vi "Test Sequencer Example.vi"() -> ()   [LabVIEW 2010]
doc: "Car Wash Main VI. Allows setup of multiple wash steps and sim of car position. Shows current step."
uses:
  Sequence Table/Sequence Table Cluster TDef.ctl
  Controls/StateMachineStates_TEST_TDEF.ctl
panel:
  out "error out":errorcluster
  out "input cluster":T1
  in  "Abort":bool
  in  "Start":bool
  in  "Pause":bool
  out "Test Running":bool
  out "Elapsed Time":dbl format="%.2g"
  in  "Test Table":string[][](table)=[[""]]
  out "Current Test":string[](array[string])
  in  "Stop Program":bool
  # "Test Sequence Configuration"
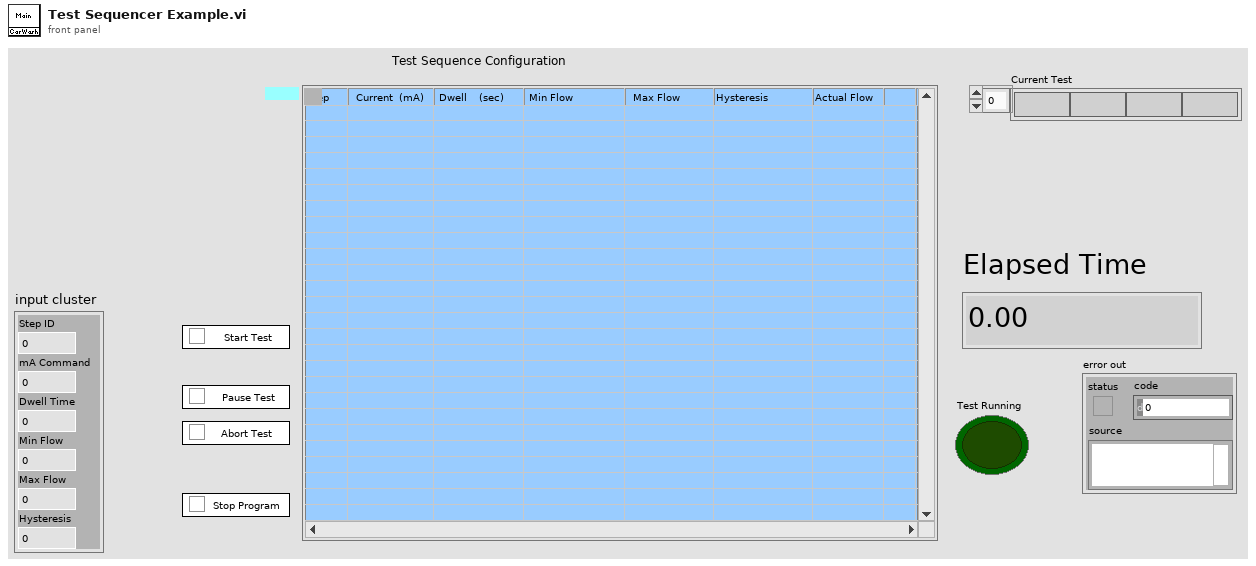
[diagram p1: front panel]
types:
  T1 = typedef "Sequence Table Cluster TDef.ctl" = cluster{"Step ID":i32, "mA Command":dbl, "Dwell Time":dbl, "Min Flow":dbl, "Max Flow":dbl, "Hysteresis":dbl}
  T2 = typedef "StateMachineStates_TEST_TDEF.ctl" = enum16{"Initialize", "Start", "Run Position", "Pause", "Resume", "Get Step"}
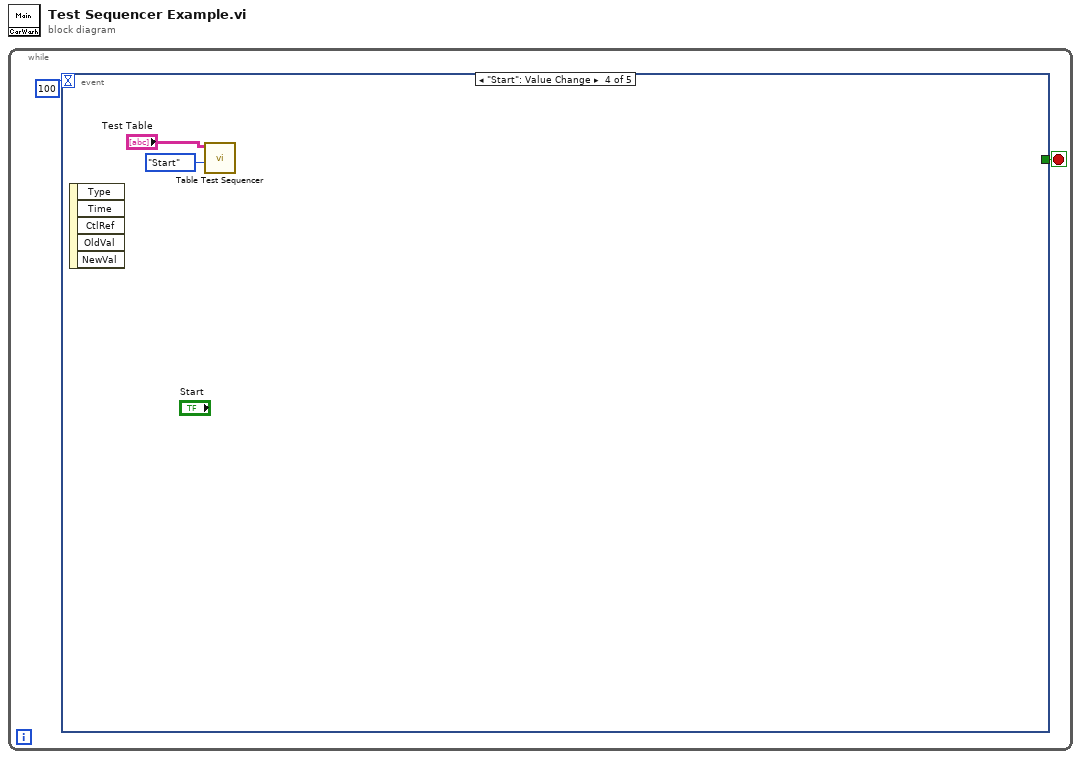
[diagram p0: block diagram]
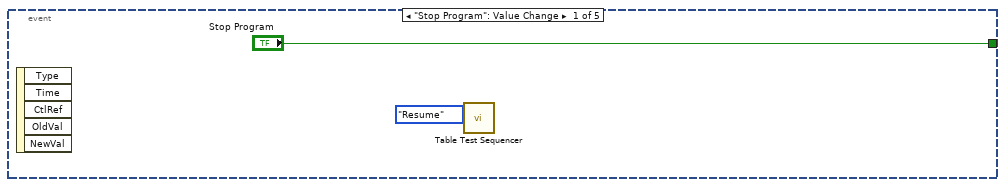
[diagram p2: hidden frame]
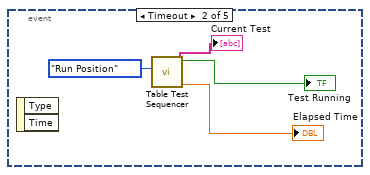
[diagram p3: hidden frame]
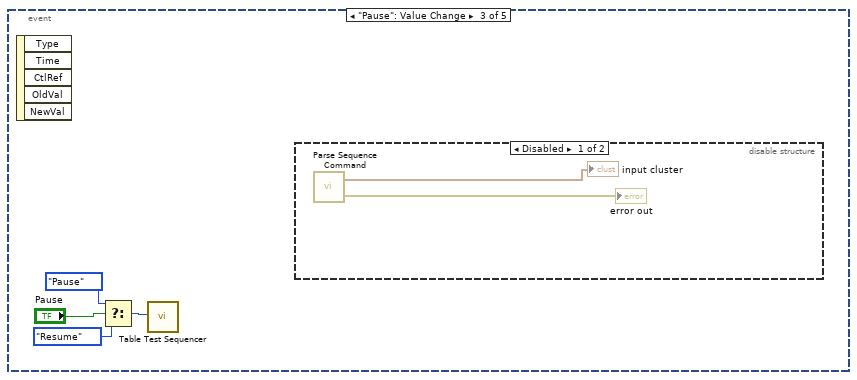
[diagram p4: hidden frame]
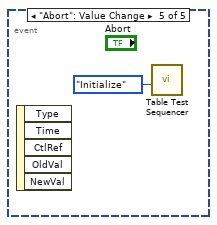
[diagram p6: hidden frame]
diagram:
  n1 = while {
    stop <- w2 stop-if-true
    n2 = event shown="[3] \"Start\": Value Change" {
      selector: _ -> [_ _ _ _ _]
      dyn-events: _ -> [_ _ _ _ _]
      timeout: 100 -> [_ _ _ _ _]
      tunnel: ["Stop Program" _ _ _ _] -> w2
      event "Stop Program": Value Change {
        n3 = event-data() -> ()  [unwired: 1 in, 5 out]
        n4 = call "Table Test Sequencer.vi"("Action"=StateMachineStates_TEST_TDEF."Resume") -> ()  [unwired: 3 in, 8 out]
      }
      event Timeout {
        n5 = event-data() -> ()  [unwired: 1 in, 2 out]
        n6 = call "Table Test Sequencer.vi"("Action"=StateMachineStates_TEST_TDEF."Run Position") -> ("Current Elapsed"=→"Elapsed Time":dbl, "Test Running"=→"Test Running":bool, "Current Test"=→"Current Test":string[])  [unwired: 3 in, 5 out]
      }
      event "Pause": Value Change {
        n7 = event-data() -> ()  [unwired: 1 in, 5 out]
        n8 = Select(t=StateMachineStates_TEST_TDEF."Pause" ("Action"), s="Pause", f=StateMachineStates_TEST_TDEF."Resume") -> (s? t:f=w9:T2)
        n9 = call "Table Test Sequencer.vi"("Action"=w9) -> ()  [unwired: 3 in, 8 out]
        n10 = disable-structure shown="Disabled" {
          frame Disabled {
            n11 = call "Parse Sequence Command.vi"() -> ("error out"=→"error out":errorcluster, "input cluster"=→"input cluster":T1)  [unwired: 1 in]
          }
          frame Enabled {
          }
        }
      }
      event "Start": Value Change {
        n12 = event-data() -> ()  [unwired: 1 in, 5 out]
        n13 = call "Table Test Sequencer.vi"("Action"=StateMachineStates_TEST_TDEF."Start", "Test Table"="Test Table") -> ()  [unwired: 2 in, 8 out]
      }
      event "Abort": Value Change {
        n14 = event-data() -> ()  [unwired: 1 in, 5 out]
        n15 = call "Table Test Sequencer.vi"("Action"=StateMachineStates_TEST_TDEF."Initialize") -> ()  [unwired: 3 in, 8 out]
      }
    }
  }
